vi "Func-엑셀 데이터를 그래프로 출력.vi"() -> ()   [LabVIEW 2015] (continued)
3.3\t9.739\n3.3\t3.3\t9.743\n3.3\t3.3\t9.744\n3.3\t3.3\t9.746\n3.3\t3.3\t9.745\n3.3\t3.3\t9.748\n3.3\t3.3\t9.753\n3.3\t3.3\t9.755\n3.3\t3.3\t9.759\n3.3\t3.3\t9.759\n3.3\t3.3\t9.762\n3.3\t3.3\t9.764\n3.3\t3.3\t9.768\n3.3\t3.3\t9.769\n3.3\t3.3\t9.769\n3.3\t3.3\t9.774\n3.3\t3.3\t9.779\n3.3\t3.3\t9.783\n3.3\t3.3\t9.784\n3.3\t3.3\t9.789\n3.3\t3.3\t9.791\n3.3\t3.3\t9.795\n3.3\t3.3\t9.798\n3.3\t3.3\t9.801\n3.3\t3.3\t9.808\n3.3\t3.3\t9.812\n3.3\t3.3\t9.821\n3.3\t3.3\t9.821\n3.3\t3.3\t9.822\n3.3\t3.3\t9.826\n3.3\t3.3\t9.823\n3.3\t3.3\t9.826\n3.3\t3.3\t9.829\n3.3\t3.3\t9.833\n3.3\t3.3\t9.835\n3.3\t3.3\t9.837\n3.3\t3.3\t9.844\n3.3\t3.3\t9.844\n3.3\t3.3\t9.844\n3.3\t3.3\t9.846\n3.3\t3.3\t9.846\n3.3\t3.3\t9.847\n3.3\t3.3\t9.846\n3.3\t3.3\t9.85\n3.3\t3.3\t9.854\n3.3\t3.3\t9.856\n3.3\t3.3\t9.865\n3.3\t3.3\t9.87\n3.3\t3.3\t9.875\n3.3\t3.3\t9.879\n3.3\t3.3\t9.883\n3.3\t3.3\t9.887\n3.3\t3.3\t9.885\n3.3\t3.3\t9.889\n3.3\t3.3\t9.892\n3.3\t3.3\t9.894\n3.3\t3.3\t9.896\n3.3\t3.3\t9.898\n3.3\t3.3\t9.9\n3.3\t3.3\t9.905\n3.3\t3.3\t9.91\n3.3\t3.3\t9.911\n3.3\t3.3\t9.915\n3.3\t3.3\t9.916\n3.3\t3.3\t9.919\n3.3\t3.3\t9.922\n3.3\t3.3\t9.923\n3.3\t3.3\t9.926\n3.3\t3.3\t9.933\n3.3\t3.3\t9.935\n3.3\t3.3\t9.939\n3.3\t3.3\t9.938\n3.3\t3.3\t9.939\n3.3\t3.3\t9.943\n3.3\t3.3\t9.945\n3.3\t3.3\t9.948\n3.3\t3.3\t9.95\n3.3\t3.3\t9.955\n3.3\t3.3\t9.956\n3.3\t3.3\t9.956\n3.3\t3.3\t9.961\n3.3\t3.3\t9.966\n3.3\t3.3\t9.966\n3.3\t3.3\t9.97\n3.3\t3.3\t9.975\n3.3\t3.3\t9.976\n3.3\t3.3\t9.977\n3.3\t3.3\t9.979\n3.3\t3.3\t9.985\n3.3\t3.3\t9.988\n3.3\t3.3\t9.991\n3.3\t3.3\t9.991\n3.3\t3.3\t9.993\n3.3\t3.3\t9.993\n3.3\t3.3\t9.992\n3.3\t3.3\t9.997\n3.3\t3.3\t9.998\n3.3\t3.3\t9.999\n3.3\t3.3\t10.006\n3.3\t3.3\t10.01\n3.3\t3.3\t10.012\n3.3\t3.3\t10.016\n3.3\t3.3\t10.021\n3.3\t3.3\t10.025\n3.3\t3.3\t10.032\n3.3\t3.3\t10.034\n3.3\t3.3\t10.038\n3.3\t3.3\t10.04\n3.3\t3.3\t10.038\n3.3\t3.3\t10.039\n3.3\t3.3\t10.035\n3.3\t3.3\t10.036\n3.3\t3.3\t10.036\n3.3\t3.3\t10.038\n3.3\t3.3\t10.042\n3.3\t3.3\t10.05\n3.3\t3.3\t10.056\n3.3\t3.3\t10.062\n3.3\t3.3\t10.062\n3.3\t3.3\t10.066\n3.3\t3.3\t10.071\n3.3\t3.3\t10.071\n3.3\t3.3\t10.071\n3.3\t3.3\t10.071\n3.3\t3.3\t10.079\n3.3\t3.3\t10.077\n3.3\t3.3\t10.076\n3.3\t3.3\t10.078\n3.3\t3.3\t10.08\n3.3\t3.3\t10.083\n3.3\t3.3\t10.086\n3.3\t3.3\t10.092\n3.3\t3.3\t10.096\n3.3\t3.3\t10.1\n3.3\t3.3\t10.103\n3.3\t3.3\t10.104\n3.3\t3.3\t10.104\n3.3\t3.3\t10.106\n3.3\t3.3\t10.106\n3.3\t3.3\t10.111\n3.3\t3.3\t10.115\n3.3\t3.3\t10.119\n3.3\t3.3\t10.121\n3.3\t3.3\t10.118\n3.3\t3.3\t10.123\n3.3\t3.3\t10.127\n3.3\t3.3\t10.126\n3.3\t3.3\t10.129\n3.3\t3.3\t10.132\n3.3\t3.3\t10.139\n3.3\t3.3\t10.14\n3.3\t3.3\t10.139\n3.3\t3.3\t10.143\n3.3\t3.3\t10.141\n3.3\t3.3\t10.147\n3.3\t3.3\t10.15\n3.3\t3.3\t10.151\n3.3\t3.3\t10.156\n3.3\t3.3\t10.159\n3.3\t3.3\t10.163\n3.3\t3.3\t10.162\n3.3\t3.3\t10.164\n3.3\t3.3\t10.166\n3.3\t3.3\t10.172\n3.3\t3.3\t10.174\n3.3\t3.3\t10.177\n3.3\t3.3\t10.183\n3.3\t3.3\t10.186\n3.3\t3.3\t10.188\n3.3\t3.3\t10.188\n3.3\t3.3\t10.192\n3.3\t3.3\t10.196\n3.3\t3.3\t10.193\n3.3\t3.3\t10.195\n3.3\t3.3\t10.197\n3.3\t3.3\t10.202\n3.3\t3.3\t10.204\n3.3\t3.3\t10.204\n3.3\t3.3\t10.209\n3.3\t3.3\t10.213\n3.3\t3.3\t10.217\n3.3\t3.3\t10.22\n3.3\t3.3\t10.222\n3.3\t3.3\t10.224\n3.3\t3.3\t10.232\n3.3\t3.3\t10.232\n3.3\t3.3\t10.231\n3.3\t3.3\t10.231\n3.3\t3.3\t10.232\n3.3\t3.3\t10.234\n3.3\t3.3\t10.233\n3.3\t3.3\t10.232\n3.3\t3.3\t10.237\n3.3\t3.3\t10.239\n3.3\t3.3\t10.241\n3.3\t3.3\t10.243\n3.3\t3.3\t10.244\n3.3\t3.3\t10.249\n3.3\t3.3\t10.25\n3.3\t3.3\t10.255\n3.3\t3.3\t10.255\n3.3\t3.3\t10.254\n3.3\t3.3\t10.259\n3.3\t3.3\t10.261\n3.3\t3.3\t10.263\n3.3\t3.3\t10.266\n3.3\t3.3\t10.269\n3.3\t3.3\t10.275\n3.3\t3.3\t10.278\n3.3\t3.3\t10.283\n3.3\t3.3\t10.287\n3.3\t3.3\t10.284\n3.3\t3.3\t10.284\n3.3\t3.3\t10.287\n3.3\t3.3\t10.288\n3.3\t3.3\t10.287\n3.3\t3.3\t10.289\n3.3\t3.3\t10.296\n3.3\t3.3\t10.302\n3.3\t3.3\t10.303\n3.3\t3.3\t10.307\n3.3\t3.3\t10.308\n3.3\t3.3\t10.31\n3.3\t3.3\t10.314\n3.3\t3.3\t10.316\n3.3\t3.3\t10.319\n3.3\t3.3\t10.32\n3.3\t3.3\t10.323\n3.3\t3.3\t10.326\n3.3\t3.3\t10.322\n3.3\t3.3\t10.324\n3.3\t3.3\t10.328\n3.3\t3.3\t10.328\n3.3\t3.3\t10.33\n3.3\t3.3\t10.334\n3.3\t3.3\t10.338\n3.3\t3.3\t10.34\n3.3\t3.3\t10.344\n3.3\t3.3\t10.348\n3.3\t3.3\t10.348\n3.3\t3.3\t10.35\n3.3\t3.3\t10.35\n3.3\t3.3\t10.352\n3.3\t3.3\t10.352\n3.3\t3.3\t10.354\n3.3\t3.3\t10.354\n3.3\t3.3\t10.355\n3.3\t3.3\t10.355\n3.3\t3.3\t10.355\n3.3\t3.3\t10.36\n3.3\t3.3\t10.361\n3.3\t3.3\t10.366\n3.3\t3.3\t10.368\n3.3\t3.3\t10.375\n3.3\t3.3\t10.377\n3.3\t3.3\t10.374\n3.3\t3.3\t10.375\n3.3\t3.3\t10.375\n3.3\t3.3\t10.381\n3.3\t3.3\t10.386\n3.3\t3.3\t10.387\n3.3\t3.3\t10.396\n3.3\t3.3\t10.398\n3.3\t3.3\t10.404\n3.3\t3.3\t10.401\n3.3\t3.3\t10.398\n3.3\t3.3\t10.401\n3.3\t3.3\t10.401\n3.3\t3.3\t10.403\n3.3\t3.3\t10.403\n3.3\t3.3\t10.408\n3.3\t3.3\t10.412\n3.3\t3.3\t10.416\n3.3\t3.3\t10.416\n3.3\t3.3\t10.419\n3.3\t3.3\t10.42\n3.3\t3.3\t10.421\n3.3\t3.3\t10.422\n3.3\t3.3\t10.427\n3.3\t3.3\t10.431\n3.3\t3.3\t10.432\n3.3\t3.3\t10.433\n3.3\t3.3\t10.438\n3.3\t3.3\t10.441\n3.3\t3.3\t10.441\n3.3\t3.3\t10.442\n3.3\t3.3\t10.445\n3.3\t3.3\t10.451\n3.3\t3.3\t10.455\n3.3\t3.3\t10.459\n3.3\t3.3\t10.458\n3.3\t3.3\t10.462\n3.3\t3.3\t10.463\n3.3\t3.3\t10.463\n3.3\t3.3\t10.462\n3.3\t3.3\t10.462\n3.3\t3.3\t10.467\n3.3\t3.3\t10.47\n3.3\t3.3\t10.47\n3.3\t3.3\t10.47\n3.3\t3.3\t10.474\n3.3\t3.3\t10.477\n3.3\t3.3\t10.474\n3.3\t3.3\t10.478\n3.3\t3.3\t10.484\n3.3\t3.3\t10.492\n3.3\t3.3\t10.494\n3.3\t3.3\t10.494\n3.3\t3.3\t10.498\n3.3\t3.3\t10.495\n3.3\t3.3\t10.493\n3.3\t3.3\t10.495\n3.3\t3.3\t10.496\n3.3\t3.3\t10.5\n3.3\t3.3\t10.504\n3.3\t3.3\t10.507\n3.3\t3.3\t10.508\n3.3\t3.3\t10.511\n3.3\t3.3\t10.514\n3.3\t3.3\t10.515\n3.3\t3.3\t10.521\n3.3\t3.3\t10.525\n3.3\t3.3\t10.528\n3.3\t3.3\t10.529\n3.3\t3.3\t10.53\n3.3\t3.3\t10.529\n3.3\t3.3\t10.53\n3.3\t3.3\t10.529\n3.3\t3.3\t10.527\n3.3\t3.3\t10.526\n3.3\t3.3\t10.531\n3.3\t3.3\t10.533\n3.3\t3.3\t10.536\n3.3\t3.3\t10.538\n3.3\t3.3\t10.542\n3.3\t3.3\t10.548\n3.3\t3.3\t10.548\n3.3\t3.3\t10.55\n3.3\t3.3\t10.551\n3.3\t3.3\t10.55\n3.3\t3.3\t10.554\n3.3\t3.3\t10.555\n3.3\t3.3\t10.557\n3.3\t3.3\t10.557\n3.3\t3.3\t10.561\n3.3\t3.3\t10.566\n3.3\t3.3\t10.567\n3.3\t3.3\t10.566\n3.3\t3.3\t10.566\n3.3\t3.3\t10.57\n3.3\t3.3\t10.57\n3.3\t3.3\t10.573\n3.3\t3.3\t10.577\n3.3\t3.3\t10.583\n3.3\t3.3\t10.586\n3.3\t3.3\t10.589\n3.3\t3.3\t10.591\n3.3\t3.3\t10.591\n3.3\t3.3\t10.591\n3.3\t3.3\t10.59\n3.3\t3.3\t10.589\n3.3\t3.3\t10.591\n3.3\t3.3\t10.597\n3.3\t3.3\t10.596\n3.3\t3.3\t10.598\n3.3\t3.3\t10.601\n3.3\t3.3\t10.604\n3.3\t3.3\t10.602\n3.3\t3.3\t10.6\n3.3\t3.3\t10.603\n3.3\t3.3\t10.604\n3.3\t3.3\t10.609\n3.3\t3.3\t10.613\n3.3\t3.3\t10.617\n3.3\t3.3\t10.619\n3.3\t3.3\t10.62\n3.3\t3.3\t10.625\n3.3\t3.3\t10.625\n3.3\t3.3\t10.626\n3.3\t3.3\t10.629\n3.3\t3.3\t10.631\n3.3\t3.3\t10.634\n3.3\t3.3\t10.632\n3.3\t3.3\t10.634\n3.3\t3.3\t10.635\n3.3\t3.3\t10.633\n3.3\t3.3\t10.636\n3.3\t3.3\t10.635\n3.3\t3.3\t10.639\n3.3\t3.3\t10.64\n3.3\t3.3\t10.639\n3.3\t3.3\t10.642\n3.3\t3.3\t10.643\n3.3\t3.3\t10.648\n3.3\t3.3\t10.65\n3.3\t3.3\t10.653\n3.3\t3.3\t10.655\n3.3\t3.3\t10.66\n3.3\t3.3\t10.663\n3.3\t3.3\t10.665\n3.3\t3.3\t10.663\n3.3\t3.3\t10.663\n3.3\t3.3\t10.667\n3.3\t3.3\t10.668\n3.3\t3.3\t10.669\n3.3\t3.3\t10.667\n3.3\t3.3\t10.673\n3.3\t3.3\t10.675\n3.3\t3.3\t10.677\n3.3\t3.3\t10.677\n3.3\t3.3\t10.678\n3.3\t3.3\t10.679\n3.3\t3.3\t10.682\n3.3\t3.3\t10.685\n3.3\t3.3\t10.686\n3.3\t3.3\t10.69\n3.3\t3.3\t10.69\n3.3\t3.3\t10.694\n3.3\t3.3\t10.694\n3.3\t3.3\t10.696\n3.3\t3.3\t10.697\n3.3\t3.3\t10.699\n3.3\t3.3\t10.702\n3.3\t3.3\t10.704\n3.3\t3.3\t10.704\n3.3\t3.3\t10.707\n3.3\t3.3\t10.706\n3.3\t3.3\t10.708\n3.3\t3.3\t10.709\n3.3\t3.3\t10.713\n3.3\t3.3\t10.716\n3.3\t3.3\t10.716\n3.3\t3.3\t10.725\n3.3\t3.3\t10.725\n3.3\t3.3\t10.727\n3.3\t3.3\t10.727\n3.3\t3.3\t10.729\n3.3\t3.3\t10.728\n3.3\t3.3\t10.723\n3.3\t3.3\t10.725\n3.3\t3.3\t10.725\n3.3\t3.3\t10.725\n3.3\t3.3\t10.726\n3.3\t3.3\t10.73\n3.3\t3.3\t10.733\n3.3\t3.3\t10.736\n3.3\t3.3\t10.738\n3.3\t3.3\t10.74\n3.3\t3.3\t10.743\n3.3\t3.3\t10.741\n3.3\t3.3\t10.745\n3.3\t3.3\t10.746\n3.3\t3.3\t10.75\n3.3\t3.3\t10.755\n3.3\t3.3\t10.755\n3.3\t3.3\t10.757\n3.3\t3.3\t10.756\n3.3\t3.3\t10.759\n3.3\t3.3\t10.759\n3.3\t3.3\t10.759\n3.3\t3.3\t10.761\n3.3\t3.3\t10.761\n3.3\t3.3\t10.77\n3.3\t3.3\t10.769\n3.3\t3.3\t10.769\n3.3\t3.3\t10.77\n3.3\t3.3\t10.773\n3.3\t3.3\t10.777\n3.3\t3.3\t10.774\n3.3\t3.3\t10.775\n3.3\t3.3\t10.776\n3.3\t3.3\t10.779\n3.3\t3.3\t10.779\n3.3\t3.3\t10.78\n3.3\t3.3\t10.785\n3.3\t3.3\t10.785\n3.3\t3.3\t10.79\n3.3\t3.3\t10.792\n3.3\t3.3\t10.794\n3.3\t3.3\t10.793\n3.3\t3.3\t10.792\n3.3\t3.3\t10.794\n3.3\t3.3\t10.796\n3.3\t3.3\t10.802\n3.3\t3.3\t10.803\n3.3\t3.3\t10.807\n3.3\t3.3\t10.81\n3.3\t3.3\t10.813\n3.3\t3.3\t10.811\n3.3\t3.3\t10.814\n3.3\t3.3\t10.814\n3.3\t3.3\t10.815\n3.3\t3.3\t10.818\n3.3\t3.3\t10.82\n3.3\t3.3\t10.821\n3.3\t3.3\t10.82\n3.3\t3.3\t10.82\n3.3\t3.3\t10.82\n3.3\t3.3\t10.823\n3.3\t3.3\t10.821\n3.3\t3.3\t10.823\n3.3\t3.3\t10.826\n3.3\t3.3\t10.83\n3.3\t3.3\t10.834\n3.3\t3.3\t10.835\n3.3\t3.3\t10.839\n3.3\t3.3\t10.843\n3.3\t3.3\t10.842\n3.3\t3.3\t10.841\n3.3\t3.3\t10.843\n3.3\t3.3\t10.846\n3.3\t3.3\t10.845\n3.3\t3.3\t10.845\n3.3\t3.3\t10.849\n3.3\t3.3\t10.855\n3.3\t3.3\t10.855\n3.3\t3.3\t10.857\n3.3\t3.3\t10.861\n3.3\t3.3\t10.864\n3.3\t3.3\t10.868\n3.3\t3.3\t10.865\n3.3\t3.3\t10.868\n3.3\t3.3\t10.868\n3.3\t3.3\t10.868\n3.3\t3.3\t10.867\n3.3\t3.3\t10.868\n3.3\t3.3\t10.87\n3.3\t3.3\t10.87\n3.3\t3.3\t10.871\n3.3\t3.3\t10.873\n3.3\t3.3\t10.874\n3.3\t3.3\t10.873\n3.3\t3.3\t10.872\n3.3\t3.3\t10.872\n3.3\t3.3\t10.874\n3.3\t3.3\t10.875\n3.3\t3.3\t10.877\n3.3\t3.3\t10.88\n3.3\t3.3\t10.886\n3.3\t3.3\t10.891\n3.3\t3.3\t10.893\n3.3\t3.3\t10.893\n3.3\t3.3\t10.896\n3.3\t3.3\t10.897\n3.3\t3.3\t10.896\n3.3\t3.3\t10.898\n3.3\t3.3\t10.898\n3.3\t3.3\t10.902\n3.3\t3.3\t10.9\n3.3\t3.3\t10.899\n3.3\t3.3\t10.9\n3.3\t3.3\t10.9\n3.3\t3.3\t10.901\n3.3\t3.3\t10.899\n3.3\t3.3\t10.902\n3.3\t3.3\t10.91\n3.3\t3.3\t10.913\n3.3\t3.3\t10.909\n3.3\t3.3\t10.909\n3.3\t3.3\t10.912\n3.3\t3.3\t10.915\n3.3\t3.3\t10.916\n3.3\t3.3\t10.914\n3.3\t3.3\t10.923\n3.3\t3.3\t10.925\n3.3\t3.3\t10.926\n3.3\t3.3\t10.929\n3.3\t3.3\t10.927\n3.3\t3.3\t10.931\n3.3\t3.3\t10.932\n3.3\t3.3\t10.932\n3.3\t3.3\t10.934\n3.3\t3.3\t10.932\n3.3\t3.3\t10.932\n3.3\t3.3\t10.931\n3.3\t3.3\t10.929\n3.3\t3.3\t10.932\n3.3\t3.3\t10.935\n3.3\t3.3\t10.939\n3.3\t3.3\t10.942\n3.3\t3.3\t10.942\n3.3\t3.3\t10.948\n3.3\t3.3\t10.952\n3.3\t3.3\t10.952\n3.3\t3.3\t10.951\n3.3\t3.3\t10.95\n3.3\t3.3\t10.953\n3.3\t3.3\t10.954\n3.3\t3.3\t10.955\n3.3\t3.3\t10.954\n3.3\t3.3\t10.954\n3.3\t3.3\t10.957\n3.3\t3.3\t10.96\n3.3\t3.3\t10.961\n3.3\t3.3\t10.959\n3.3\t3.3\t10.963\n3.3\t3.3\t10.966\n3.3\t3.3\t10.965\n3.3\t3.3\t10.964\n3.3\t3.3\t10.964\n3.3\t3.3\t10.967\n3.3\t3.3\t10.971\n3.3\t3.3\t10.974\n3.3\t3.3\t10.976\n3.3\t3.3\t10.979\n3.3\t3.3\t10.98\n3.3\t3.3\t10.981\n3.3\t3.3\t10.977\n3.3\t3.3\t10.978\n3.3\t3.3\t10.98\n3.3\t3.3\t10.984\n3.3\t3.3\t10.987\n3.3\t3.3\t10.991\n3.3\t3.3\t10.995\n3.3\t3.3\t10.994\n3.3\t3.3\t10.995\n3.3\t3.3\t10.993\n3.3\t3.3\t10.996\n3.3\t3.3\t10.991\n3.3\t3.3\t10.993\n3.3\t3.3\t10.998\n3.3\t3.3\t10.999\n3.3\t3.3\t11.002\n3.3\t3.3\t11.004\n3.3\t3.3\t11.005\n3.3\t3.3\t11.004\n3.3\t3.3\t11.007\n3.3\t3.3\t11.01\n3.3\t3.3\t11.011\n3.3\t3.3\t11.013\n3.3\t3.3\t11.02\n3.3\t3.3\t11.02\n3.3\t3.3\t11.024\n3.3\t3.3\t11.021\n3.3\t3.3\t11.021\n3.3\t3.3\t11.02\n3.3\t3.3\t11.016\n3.3\t3.3\t11.018\n3.3\t3.3\t11.017\n3.3\t3.3\t11.022\n3.3\t3.3\t11.023\n3.3\t3.3\t11.024\n3.3\t3.3\t11.029\n3.3\t3.3\t11.031\n3.3\t3.3\t11.032\n3.3\t3.3\t11.033\n3.3\t3.3\t11.033\n3.3\t3.3\t11.034\n3.3\t3.3\t11.036\n3.3\t3.3\t11.038\n3.3\t3.3\t11.04\n3.3\t3.3\t11.04\n3.3\t3.3\t11.042\n3.3\t3.3\t11.042\n3.3\t3.3\t11.042\n3.3\t3.3\t11.045\n3.3\t3.3\t11.046\n3.3\t3.3\t11.048\n3.3\t3.3\t11.052\n3.3\t3.3\t11.059\n3.3\t3.3\t11.061\n3.3\t3.3\t11.057\n3.3\t3.3\t11.062\n3.3\t3.3\t11.058\n3.3\t3.3\t11.057\n3.3\t3.3\t11.057\n3.3\t3.3\t11.055\n3.3\t3.3\t11.056\n3.3\t3.3\t11.058\n3.3\t3.3\t11.062\n3.3\t3.3\t11.064\n3.3\t3.3\t11.064\n3.3\t3.3\t11.069\n3.3\t3.3\t11.073\n3.3\t3.3\t11.073\n3.3\t3.3\t11.073\n3.3\t3.3\t11.075\n3.3\t3.3\t11.08\n3.3\t3.3\t11.08\n3.3\t3.3\t11.078\n3.3\t3.3\t11.08\n3.3\t3.3\t11.08\n3.3\t3.3\t11.079\n3.3\t3.3\t11.077\n3.3\t3.3\t11.077\n3.3\t3.3\t11.084\n3.3\t3.3\t11.086\n3.3\t3.3\t11.091\n3.3\t3.3\t11.096\n3.3\t3.3\t11.092\n3.3\t3.3\t11.095\n3.3\t3.3\t11.091\n3.3\t3.3\t11.09\n3.3\t3.3\t11.089\n3.3\t3.3\t11.089\n3.3\t3.3\t11.095\n3.3\t3.3\t11.094\n3.3\t3.3\t11.097\n3.3\t3.3\t11.098\n3.3\t3.3\t11.1\n3.3\t3.3\t11.102\n3.3\t3.3\t11.101\n3.3\t3.3\t11.104\n3.3\t3.3\t11.107\n3.3\t3.3\t11.108\n3.3\t3.3\t11.109\n3.3\t3.3\t11.112\n3.3\t3.3\t11.115\n3.3\t3.3\t11.115\n3.3\t3.3\t11.116\n3.3\t3.3\t11.118\n3.3\t3.3\t11.12\n3.3\t3.3\t11.12\n3.3\t3.3\t11.123\n3.3\t3.3\t11.123\n3.3\t3.3\t11.125\n3.3\t3.3\t11.127\n3.3\t3.3\t11.129\n3.3\t3.3\t11.132\n3.3\t3.3\t11.132\n3.3\t3.3\t11.135\n3.3\t3.3\t11.13\n3.3\t3.3\t11.13\n3.3\t3.3\t11.127\n3.3\t3.3\t11.127\n3.3\t3.3\t11.128\n3.3\t3.3\t11.127\n3.3\t3.3\t11.136\n3.3\t3.3\t11.139\n3.3\t3.3\t11.141\n3.3\t3.3\t11.139\n3.3\t3.3\t11.139\n3.3\t3.3\t11.14\n3.3\t3.3\t11.14\n3.3\t3.3\t11.14\n3.3\t3.3\t11.14\n3.3\t3.3\t11.145\n3.3\t3.3\t11.146\n3.3\t3.3\t11.15\n3.3\t3.3\t11.15\n3.3\t3.3\t11.149\n3.3\t3.3\t11.152\n3.3\t3.3\t11.153\n3.3\t3.3\t11.154\n3.3\t3.3\t11.152\n3.3\t3.3\t11.156\n3.3\t3.3\t11.156\n3.3\t3.3\t11.155\n3.3\t3.3\t11.157\n3.3\t3.3\t11.161\n3.3\t3.3\t11.163\n3.3\t3.3\t11.164\n3.3\t3.3\t11.166\n3.3\t3.3\t11.168\n3.3\t3.3\t11.164\n3.3\t3.3\t11.164\n3.3\t3.3\t11.168\n3.3\t3.3\t11.168\n3.3\t3.3\t11.174\n3.3\t3.3\t11.177\n3.3\t3.3\t11.183\n3.3\t3.3\t11.182\n3.3\t3.3\t11.184\n3.3\t3.3\t11.188\n3.3\t3.3\t11.185\n3.3\t3.3\t11.187\n3.3\t3.3\t11.186\n3.3\t3.3\t11.186\n3.3\t3.3\t11.184\n3.3\t3.3\t11.182\n3.3\t3.3\t11.182\n3.3\t3.3\t11.183\n3.3\t3.3\t11.182\n3.3\t3.3\t11.182\n3.3\t3.3\t11.184\n3.3\t3.3\t11.187\n3.3\t3.3\t11.188\n3.3\t3.3\t11.187\n3.3\t3.3\t11.191\n3.3\t3.3\t11.195\n3.3\t3.3\t11.195\n3.3\t3.3\t11.194\n3.3\t3.3\t11.194\n3.3\t3.3\t11.195\n3.3\t3.3\t11.195\n3.3\t3.3\t11.195\n3.3\t3.3\t11.196\n3.3\t3.3\t11.202\n3.3\t3.3\t11.204\n3.3\t3.3\t11.203\n3.3\t3.3\t11.202\n3.3\t3.3\t11.202\n3.3\t3.3\t11.198\n3.3\t3.3\t11.193\n3.3\t3.3\t11.191\n3.3\t3.3\t11.194\n3.3\t3.3\t11.201\n3.3\t3.3\t11.206\n3.3\t3.3\t11.211\n3.3\t3.3\t11.214\n3.3\t3.3\t11.222\n3.3\t3.3\t11.225\n3.3\t3.3\t11.224\n3.3\t3.3\t11.223\n3.3\t3.3\t11.223\n3.3\t3.3\t11.226\n3.3\t3.3\t11.223\n3.3\t3.3\t11.223\n3.3\t3.3\t11.225\n3.3\t3.3\t11.227\n3.3\t3.3\t11.227\n3.3\t3.3\t11.225\n3.3\t3.3\t11.228\n3.3\t3.3\t11.225\n3.3\t3.3\t11.228\n3.3\t3.3\t11.228\n3.3\t3.3\t11.231\n3.3\t3.3\t11.232\n3.3\t3.3\t11.229\n3.3\t3.3\t11.236\n3.3\t3.3\t11.236\n3.3\t3.3\t11.236\n3.3\t3.3\t11.238\n3.3\t3.3\t11.241\n3.3\t3.3\t11.244\n3.3\t3.3\t11.246\n3.3\t3.3\t11.25\n3.3\t3.3\t11.252\n3.3\t3.3\t11.248\n3.3\t3.3\t11.25\n3.3\t3.3\t11.251\n3.3\t3.3\t11.248\n3.3\t3.3\t11.248\n3.3\t3.3\t11.249\n3.3\t3.3\t11.251\n3.3\t3.3\t11.253\n3.3\t3.3\t11.25\n3.3\t3.3\t11.251\n3.3\t3.3\t11.251\n3.3\t3.3\t11.251\n3.3\t3.3\t11.254\n3.3\t3.3\t11.253\n3.3\t3.3\t11.255\n3.3\t3.3\t11.258\n3.3\t3.3\t11.261\n3.3\t3.3\t11.262\n3.3\t3.3\t11.264\n3.3\t3.3\t11.266\n3.3\t3.3\t11.269\n3.3\t3.3\t11.271\n3.3\t3.3\t11.273\n3.3\t3.3\t11.277\n3.3\t3.3\t11.278\n3.3\t3.3\t11.28\n3.3\t3.3\t11.283\n3.3\t3.3\t11.282\n3.383\t3.35\t11.841\n3.467\t3.42\t11.852\n3.55\t3.28\t11.85\n3.633\t3.24\t11.861\n3.717\t3.18\t11.856\n3.8\t3.11\t11.86\n3.883\t3\t11.857\n3.967\t2.87\t11.86\n4.05\t2.76\t11.867\n4.133\t2.64\t11.87\n4.217\t2.52\t11.879\n4.3\t2.41\t11.872\n4.383\t2.29\t11.879\n4.467\t2.19\t11.875\n4.55\t2.12\t11.87\n4.633\t2.06\t11.884\n4.717\t2.01\t11.881\n4.8\t1.97\t11.87\n4.883\t1.94\t11.884\n4.967\t1.93\t11.869\n5.05\t1.93\t11.874\n5.133\t1.94\t11.874\n5.217\t1.96\t11.874\n5.3\t1.99\t11.875\n5.383\t2.03\t11.869\n5.467\t2.09\t11.866\n5.55\t2.16\t11.867\n5.633\t2.23\t11.854\n5.717\t2.31\t11.85\n5.8\t2.39\t11.841\n5.883\t2.47\t11.848\n5.967\t2.57\t11.837\n6.05\t2.67\t11.835\n6.133\t2.76\t11.834\n6.217\t2.85\t11.816\n6.3\t2.95\t11.822\n6.383\t3.06\t11.817\n6.467\t3.16\t11.81\n6.55\t3.26\t11.801\n6.633\t3.36\t11.8\n6.717\t3.45\t11.792\n6.8\t3.55\t11.794\n6.883\t3.65\t11.789\n6.967\t3.75\t11.785\n7.05\t3.84\t11.782\n7.133\t3.95\t11.782\n7.217\t4.04\t11.78\n7.3\t4.12\t11.782\n7.383\t4.21\t11.776\n7.467\t4.3\t11.776\n7.55\t4.39\t11.776\n7.633\t4.48\t11.773\n7.717\t4.57\t11.775\n7.8\t4.64\t11.77\n7.883\t4.72\t11.78\n7.967\t4.8\t11.781\n8.05\t4.88\t11.786\n8.133\t4.96\t11.787\n8.217\t5.04\t11.792\n8.3\t5.12\t11.804\n8.383\t5.2\t11.802\n8.467\t5.27\t11.809\n8.55\t5.35\t11.82\n8.633\t5.44\t11.825\n8.717\t5.52\t11.833\n8.8\t5.59\t11.85\n8.883\t5.66\t11.85\n8.967\t5.73\t11.869\n9.05\t5.81\t11.873\n9.133\t5.89\t11.888\n9.217\t5.96\t11.899\n9.3\t6.03\t11.917\n9.383\t6.1\t11.93\n9.467\t6.16\t11.942\n9.55\t6.24\t11.96\n9.633\t6.32\t11.973\n9.717\t6.39\t11.988\n9.8\t6.48\t12.002\n9.883\t6.55\t12.029\n9.967\t6.63\t12.046\n10.05\t6.71\t12.063\n10.133\t6.79\t12.086\n10.217\t6.87\t12.102\n10.3\t6.94\t12.124\n10.383\t7.02\t12.138\n10.467\t7.1\t12.171\n10.55\t7.19\t12.195\n10.633\t7.27\t12.218\n10.717\t7.34\t12.23\n10.8\t7.43\t12.259\n10.883\t7.51\t12.275\n10.967\t7.59\t12.307\n11.05\t7.67\t12.333\n11.133\t7.75\t12.357\n11.217\t7.83\t12.388\n11.3\t7.91\t12.413\n11.383\t7.99\t12.437\n11.467\t8.07\t12.471\n11.55\t8.15\t12.499\n11.633\t8.22\t12.527\n11.717\t8.3\t12.56\n11.8\t8.37\t12.596\n11.883\t8.45\t12.62\n11.967\t8.54\t12.652\n12.05\t8.62\t12.679\n12.133\t8.7\t12.718\n12.217\t8.78\t12.743\n12.3\t8.86\t12.778\n12.383\t8.94\t12.814\n12.467\t9.02\t12.85\n12.55\t9.11\t12.887\n12.633\t9.19\t12.918\n12.717\t9.27\t12.954\n12.8\t9.34\t12.987\n12.883\t9.42\t13.033\n12.967\t9.5\t13.067\n13.05\t9.58\t13.1\n13.133\t9.66\t13.145\n13.217\t9.74\t13.168\n13.3\t9.82\t13.223\n13.383\t9.91\t13.248\n13.467\t9.99\t13.301\n13.55\t10.08\t13.329\n13.633\t10.15\t13.377\n13.717\t10.24\t13.409\n13.8\t10.31\t13.455\n13.883\t10.39\t13.498\n13.967\t10.47\t13.531\n14.05\t10.55\t13.578\n14.133\t10.62\t13.627\n14.217\t10.7\t13.672\n14.3\t10.77\t13.717\n14.383\t10.85\t13.753\n14.467\t10.94\t13.792\n14.55\t11.02\t13.843\n14.633\t11.1\t13.883\n14.717\t11.17\t13.931\n14.8\t11.24\t13.978\n14.883\t11.32\t14.02\n14.967\t11.39\t14.07\n15.05\t11.46\t14.109\n15.133\t11.54\t14.154\n15.217\t11.63\t14.204\n15.3\t11.71\t14.258\n15.383\t11.8\t14.299\n15.467\t11.88\t14.345\n15.55\t11.96\t14.398\n15.633\t12.05\t14.44\n15.717\t12.12\t14.493\n15.8\t12.2\t14.545\n15.883\t12.28\t14.579\n15.967\t12.35\t14.641\n16.05\t12.42\t14.683\n16.133\t12.51\t14.733\n16.217\t12.59\t14.794\n16.3\t12.67\t14.846\n16.383\t12.76\t14.898\n16.467\t12.84\t14.943\n16.55\t12.92\t14.999\n16.633\t13.01\t15.05\n16.717\t13.09\t15.103\n16.8\t13.17\t15.155\n16.883\t13.25\t15.205\n16.967\t13.33\t15.266\n17.05\t13.41\t15.317\n17.133\t13.49\t15.378\n17.217\t13.57\t15.43\n17.3\t13.65\t15.475\n17.383\t13.73\t15.531\n17.467\t13.82\t15.588\n17.55\t13.89\t15.653\n17.633\t13.98\t15.704\n17.717\t14.06\t15.757\n17.8\t14.14\t15.814\n17.883\t14.22\t15.871\n17.967\t14.3\t15.927\n18.05\t14.38\t15.988\n18.133\t14.44\t16.047\n18.217\t14.52\t16.098\n18.3\t14.6\t16.164\n18.383\t14.68\t16.222\n18.467\t14.75\t16.28\n18.55\t14.83\t16.341\n18.633\t14.91\t16.393\n18.717\t14.99\t16.453\n18.8\t15.07\t16.521\n18.883\t15.14\t16.571\n18.967\t15.23\t16.627\n19.05\t15.32\t16.687\n19.133\t15.4\t16.757\n19.217\t15.49\t16.82\n19.3\t15.57\t16.869\n19.383\t15.65\t16.946\n19.467\t15.73\t16.996\n19.55\t15.81\t17.058\n19.633\t15.88\t17.124\n19.717\t15.96\t17.186\n19.8\t16.03\t17.249\n19.883\t16.11\t17.305\n19.967\t16.19\t17.372\n20.05\t16.27\t17.425\n20.133\t16.33\t17.493\n20.217\t16.41\t17.551\n20.3\t16.49\t17.621\n20.383\t16.57\t17.689\n20.467\t16.65\t17.753\n20.55\t16.73\t17.802\n20.633\t16.81\t17.875\n20.717\t16.89\t17.937\n20.8\t16.97\t18\n20.883\t17.06\t18.062\n20.967\t17.13\t18.122\n21.05\t17.21\t18.177\n21.133\t17.29\t18.263\n21.217\t17.37\t18.311\n21.3\t17.45\t18.38\n21.383\t17.53\t18.447\n21.467\t17.6\t18.5\n21.55\t17.69\t18.571\n21.633\t17.77\t18.646\n21.717\t17.85\t18.706\n21.8\t17.94\t18.764\n21.883\t18.02\t18.838\n21.967\t18.1\t18.907\n22.05\t18.17\t
